vi "GlobalVariableS.vi"() -> ()   [LabVIEW 2017]
uses:
  TypeDef/ESC_StateMachine.ctl
panel:
  out "DEBUG notes":string
  in  "WebBrowser":refnum<k7>(container)
  out "Conversion Progress 2":dbl(slide) scale=0.0..100.0
  out "Conversion Progress 1":dbl(slide) scale=0.0..100.0
  out "Next State":T1=enum."Play File"
  out "This State":T1=enum."Play File"
  in  "Enable scaling 2":bool=TRUE
  out "JSON string":string="{\"BB_Gain\": \"5.411e-07\", \"Test_File\": \"D:\\\\FOUO\\\\1RDR1P2LTE.dat\", \"RF_Gain\": \"10\", \"RF_Center_Freq\": \"3550000000\"}"
  out "error IO":errorcluster={"status"=TRUE, "code"=363500, "source"="LabVIEWHTTPClient.lvlib:POSTBuffer.vi:6120001<APPEND>\n\n<b>Complete call chain:</b>\r\n     LabVIEWHTTPClient.lvlib:POSTBuffer.vi:6120001\r\n     ESC_Harness_InstructionsListener.vi\r\n     Main_System.vi\r\n     Main_System.vi.ProxyCaller"}
  in  "Enable scaling":bool=TRUE
  out "BB_Gain":string="5.411e-07"
  out "RF_Center_Freq":string="3550000000"
  out "RF_Gain":string="10"
  out "Error":string
  out "Status":string="Done"
  out "Test_File":string="D:\\FOUO\\1RDR1P2LTE.dat"
  out "Playback Progress":i32(slide)=-1 scale=-1.0..536.0
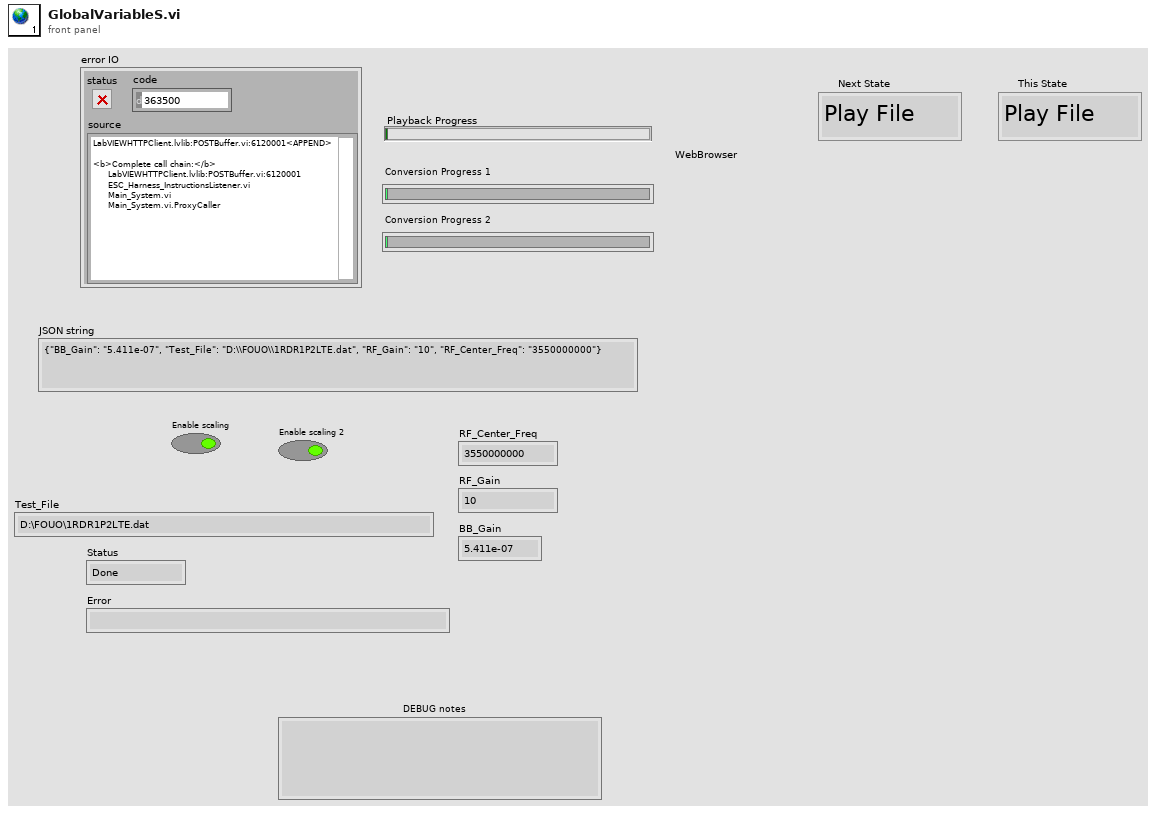
[diagram p1: front panel]
types:
  T1 = typedef "ESC_StateMachine.ctl" = enum16{"Parse Metadata", "Convert File", "Play File", "Finished Playing", "Send Message", "Report Error", "Exit"}
diagram:
